vi "Get_Source.vi"(8 "error in (no error)":errorcluster, 11 "IB_Source in":refnum<class "IB_Source.lvclass">) -> (0 "error out":errorcluster, 2 "data":T1, 3 "IB_Source out":refnum<class "IB_Source.lvclass">)   [LabVIEW 2020, in "IB_Source.lvclass"]
uses:
  <vilib>/AppBuilder/IB_Classes/Source/IB_Source.lvclass
  <vilib>/AppBuilder/IB_Classes/Source/IB_Source.lvclass/IB_Source.ctl
  <vilib>/AppBuilder/IB_Classes/Source/IB_Source.ctl
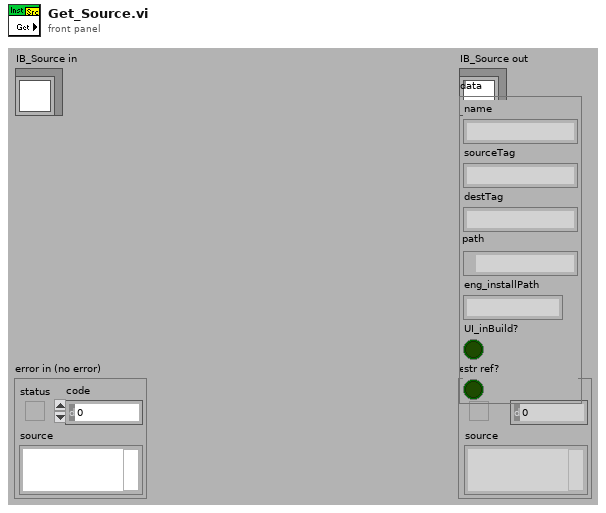
[diagram p1: front panel]
types:
  T1 = typedef "IB_Source.ctl" = cluster{"name":string, "sourceTag":string, "destTag":string, "path":path, "eng_installPath":string, "UI_inBuild?":bool, "str ref?":bool}
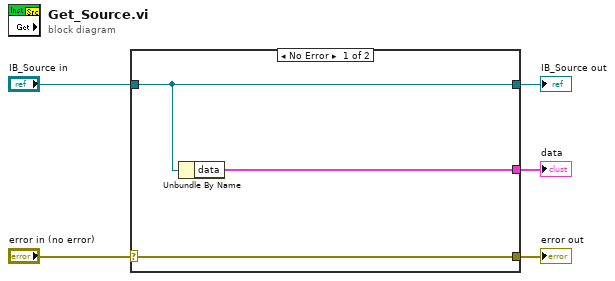
[diagram p0: block diagram]
diagram:
  n1 = case shown="No Error" "error in (no error)" {
    selector: "error in (no error)" -> [w8 w9]
    tunnel: [w8 w9] -> w4
    tunnel: [w7 w10] -> w2
    tunnel: "IB_Source in" -> [w7 w10]
    tunnel: [w6 _] -> w1
    frame No Error {
      n2 = Unbundle By Name(w7) -> ("data"=w6:T1)
    }
    frame Error {
    }
  }
  "error out" <- w4
  "IB_Source out" <- w2
  "data" <- w1
